vi "FITS Test Program.vi"() -> ()   [LabVIEW 2020]
uses:
  <userlib>/gfitsio/gfitsio-write-key-double.vi
  <userlib>/gfitsio/gfitsio.lvlib
panel:
  out "header":string[](array[string])
  in  "file path (dialog if empty)":path
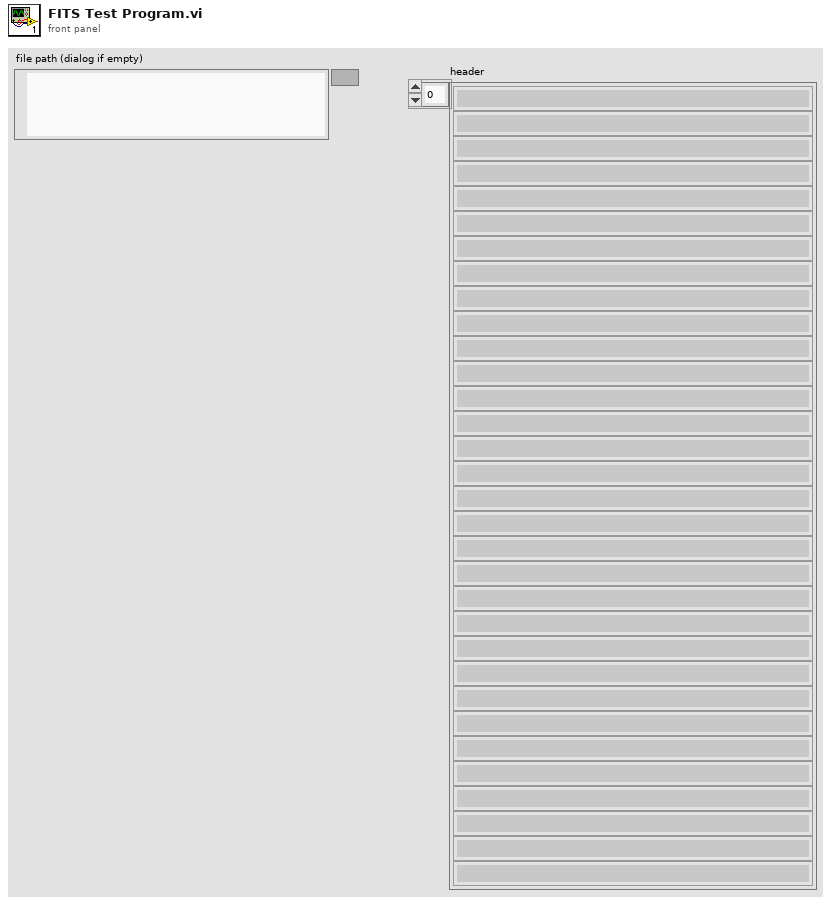
[diagram p1: front panel]
types:
  T1 = typedef "gfitsio.lvlib/gfitsio-refnum.ctl" = refnum<k1>
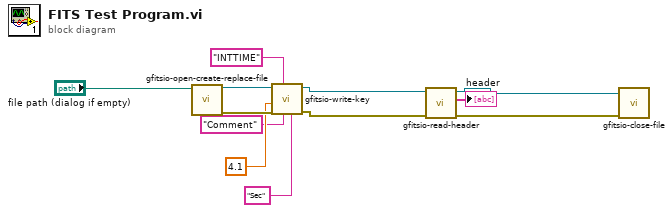
[diagram p0: block diagram]
diagram:
  n1 = call <userlib>:"gfitsio-open-create-replace-file.vi"("file path (dialog if empty)"="file path (dialog if empty)") -> ("error out"=w11:errorcluster, "gfits refnum"=w10:T1)  [unwired: 8 in, 1 out]
  n2 = call-poly <userlib>:"gfitsio-write-key.vi"("units"="Sec", "comment"="Comment", "keyname"="INTTIME", "error in (no error)"=w11, "value"=4.1, "gfits refnum"=w10) -> ("error out"=w5:errorcluster, "dup gfits refnum"=w7:T1)  [unwired: 4 in]
  n3 = call <userlib>:"gfitsio-read-header.vi"("error in (no error)"=w5, "gfits refnum"=w7) -> ("error out"=w3:errorcluster, "header"=→"header":string[], "dup gfits refnum"=w4:T1)  [unwired: 7 in]
  n4 = call <userlib>:"gfitsio-close-file.vi"("error in (no error)"=w3, "gfits refnum"=w4) -> ()  [unwired: 8 in, 2 out]
